vi "Write to Driver Station.vi"   [LabVIEW 2012]
uses:
  Globals/Useful Values.vi
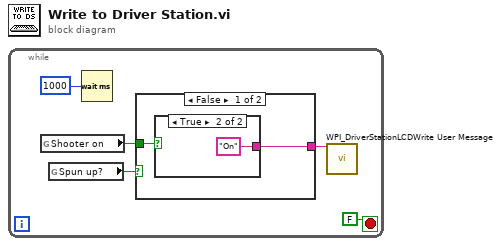
[diagram p0: block diagram]
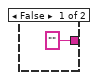
[diagram p2: hidden frame]
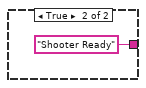
[diagram p3: hidden frame]
diagram:
  n1 = while {
    stop <- FALSE stop-if-true
    n2 = global read "Useful Values.vi" "Shooter on"() -> (w1:bool)
    n3 = global read "Useful Values.vi" "Spun up?"() -> (w3:bool)
    n4 = Wait (ms)(milliseconds to wait=u32 1000) -> ()  [unwired: 1 out]
    n5 = case shown="False" w3 {
      tunnel: [w6 "Shooter Ready" ("line text")] -> w2
      tunnel: w1 -> [w7 _]
      frame False {
        n6 = case shown="True" w7 {
          tunnel: ["" ("line text") "On" ("line text")] -> w6
          frame False {
          }
          frame True {
          }
        }
      }
      frame True {
      }
    }
    n7 = call <vilib>:"WPI_DriverStationLCDWrite User Message.vi"("line text"=w2) -> ()  [unwired: 14 in, 1 out]
  }
